vi "Set Camera Status Enable.vi"(11 "Enable":u32) -> (3 "function return":u32)   [LabVIEW 2018, in "Copy of Andor SDK.lvlib"]
doc: "EXPNETTYPE unsigned int WINAPI SetCameraStatusEnable(DWORD Enable);"
uses:
  Copy of Andor SDK.lvlib
  <userlib>/Andor SDK/ATMCD32D.dll
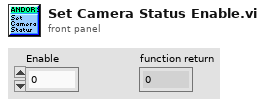
[diagram p1: front panel]
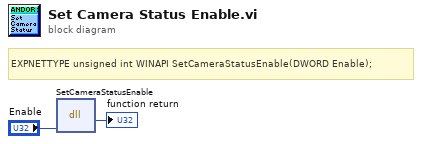
[diagram p0: block diagram]
diagram:
  # "EXPNETTYPE unsigned int WINAPI SetCameraStatusEnable(DWORD Enable);"
  n1 = dll-call lib="C:/Program Files (x86)/National Instruments/LabVIEW 2018/user.lib/Andor SDK/ATMCD32D.*" fn="SetCameraStatusEnable"("Enable"="Enable") -> (→"function return":u32)  [unwired: 4 in, 2 out]
